vi "flush.vi"(8 "error in":errorcluster, 11 "refnum in":T1) -> (0 "error out":errorcluster, 1 "flushed data[]":cluster{"Command":string, "Data":variant}[](array[cluster]), 3 "refnum out":T1)   [LabVIEW 2020, in "Publisher Subscriber.lvlib"]
doc: "Flush all the elements from the buffer for this node."
uses:
  Publisher Subscriber.lvlib
  Controls/node refnum.ctl
  Controls/node dvr data.ctl
  Controls/data cluster.ctl
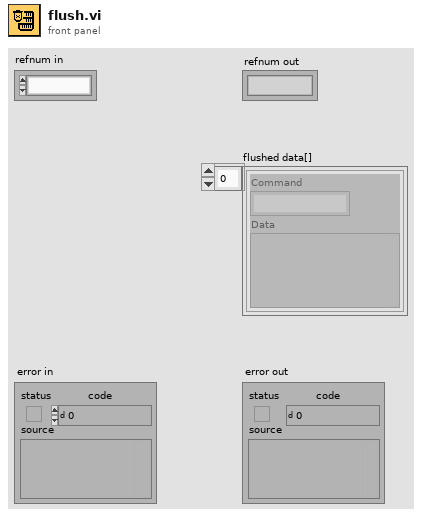
[diagram p1: front panel]
types:
  T1 = typedef "Publisher Subscriber.lvlib/node refnum.ctl" = refnum<k1>
  T2 = typedef "Publisher Subscriber.lvlib/node dvr data.ctl" = cluster{"queue ref":refnum<queue>, "subscription map ref":refnum<data-value>, "Command":string, "Data":variant, "Subscriptions []":set{string}, "variable dvr refs":refnum<data-value>}
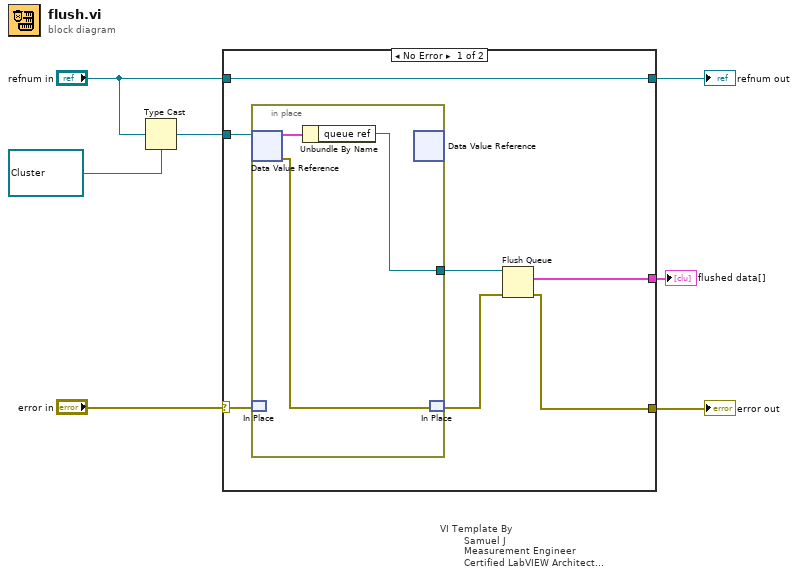
[diagram p0: block diagram]
diagram:
  n1 = Type Cast(type=refnum<data-value> refnum ("data value reference"), x="refnum in") -> (*(type *) &x=w4:refnum<data-value>)
  n2 = case "VI Template By\n        Samuel J\n        Measurement Engineer\n        Certified LabVIEW Architect\n        Vestas Technology R&D Chennai" shown="No Error" "error in" {
    selector: "error in" -> [w12 w19]
    tunnel: [w9 w19] -> w6
    tunnel: w4 -> [w13 _]
    tunnel: [w14 w18] -> w3
    tunnel: "refnum in" -> [w14 w18]
    tunnel: [w8 _] -> w1
    frame No Error {
      n3 = in-place {
        in-place-border: [w15] -> w11
        n4 = in-place-dvr #1(w13) -> (w17:T2, w16:errorcluster)
        n5 = in-place-match #2(w12) -> ()  [unwired: 1 out]
        n6 = Unbundle By Name(w17) -> ("queue ref"=w15:refnum<queue>)
        n7 = in-place-dvr #1() -> ()  [unwired: 1 in, 2 out]
        n8 = in-place-match #2(w16) -> (w10:errorcluster)
      }
      n9 = Flush Queue(queue=w11, error in (no error)=w10) -> (remaining elements=w8:cluster{"Command":string, "Data":variant}[], error out=w9:errorcluster)  [unwired: 1 out]
    }
    frame Error {
    }
  }
  "error out" <- w6
  "refnum out" <- w3
  "flushed data[]" <- w1
